vi "Start_Serving.vi"() -> ()   [LabVIEW 2022 SP3]
doc: "This is a simple example of a server which exports VIs to be called from another machine. You may run both the client.llb and server.llb on the same machine without modifying the access list. If you wish to run the client on another machine that is not in your domain you will have to list the name of the client in the Machine Access List. \n\nThe VIs listed in the Exported VI list are exported by the server.\n\nTo run this example start this VI First, then start the client.llb on all machines you want to try as clients. If you change either of the above lists, you must restart this VI for the changes to take effect.\n\nClick the \"Stop\" button to quit. This will turn off the server, terminating all client connections, and restore the previous access lists to their original values."
uses:
  Anemometry/Anemometry Sub Vis/Globals/Preference_global.vi
panel:
  out "logPath":path
  in  "Srvr.LogEnabled":bool
  out "Exported VI list":string[](array[string])
  # "These are the names of the VIs which will be allowed\nto be accessed from another machine."
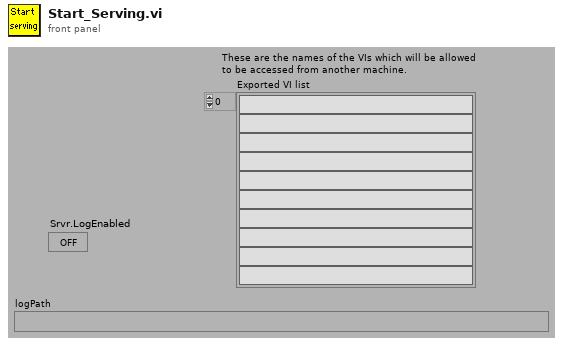
[diagram p1: front panel]
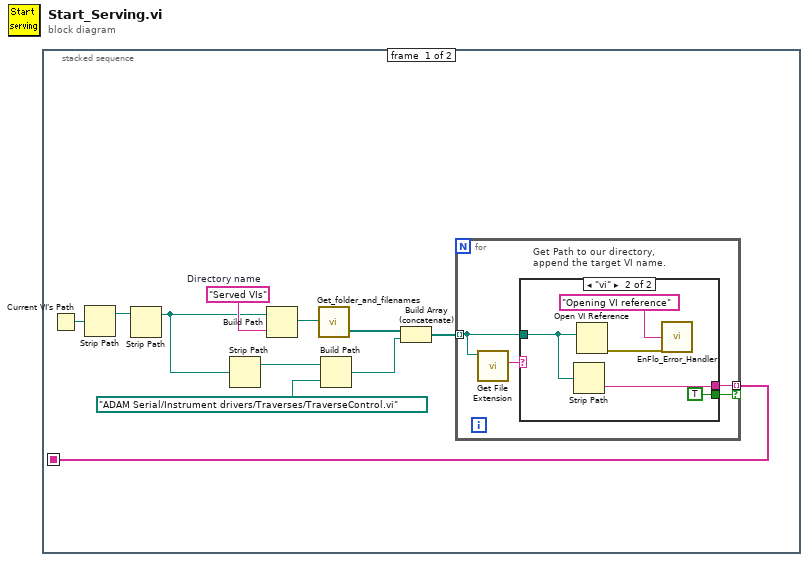
[diagram p0: block diagram]
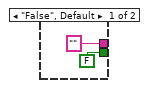
[diagram p2: hidden frame]
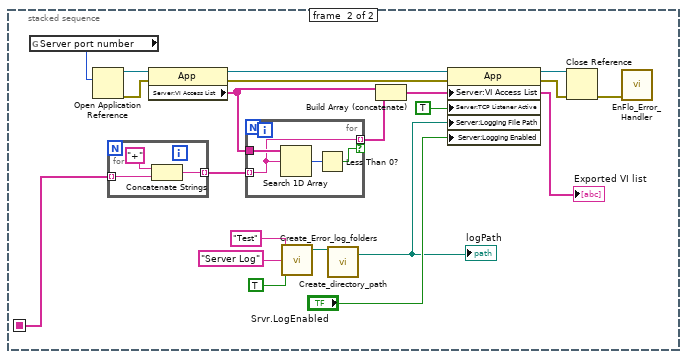
[diagram p3: hidden frame]
diagram:
  n1 = stacked-sequence {
    seq-local: [w1 _] -> [_ w26]
    frame #0 {
      w11 = "Served VIs"  # Directory name
      n2 = Current VI's Path() -> (path=w10:path)
      n3 = Strip Path(path=w10) -> (stripped path=w9:path)  [unwired: 1 out]
      n4 = Strip Path(path=w9) -> (stripped path=w7:path)  [unwired: 1 out]
      n5 = Strip Path(path=w7) -> (stripped path=w6:path)  [unwired: 1 out]
      n6 = Build Path(base path=w7, name or relative path=w11) -> (appended path=w8:path)
      n7 = call "Get_folder_and_filenames.vi"("file path (dialog if empty)"=w8) -> ("Files"=w4:path[])  [unwired: 1 out]
      n8 = Build Path(base path=w6, name or relative path=path "ADAM Serial/Instrument drivers/Traverses/TraverseControl.vi") -> (appended path=w3:path)
      n9 = Build Array (concatenate)(w4, w3) -> (w2:path[])
      n10 = for {
        tunnel: w2 -> [w14] mode=indexing
        tunnel: [w15] -> w1 mode=indexing if=w12
        # "Get Path to our directory,\nappend the target VI name."
        n11 = call <vilib>:"Get File Extension.vi"("file"=w14) -> ("lowercase file extension"=w13:string)  [unwired: 6 in, 4 out]
        n12 = case shown="\"vi\"" w13 {
          tunnel: ["" ("name") w22] -> w15
          tunnel: w14 -> [_ w19]
          tunnel: [FALSE TRUE] -> w12
          frame "False", Default {
          }
          frame "vi" {
            n13 = Strip Path(path=w19) -> (name=w22:string)  [unwired: 1 out]
            n14 = Open VI Reference(vi path=w19) -> (error out=w21:errorcluster)  [unwired: 2 in, 4 out]
            n15 = call "EnFlo_Error_Handler.vi"("error in (no error)"=w21, "Error Type"="Opening VI reference") -> ()  [unwired: 1 in, 3 out]
          }
        }
      }
    }
    frame #1 {
      n16 = global read "Preference_global.vi" "Server port number"() -> (w38:u32)
      n17 = Open Application Reference(10:w38) -> (0:w31:errorcluster, 3:w32:refnum<vi>)  [unwired: 1 in, 2 out]
      n18 = for {
        tunnel: [w44] -> w25 mode=indexing
        tunnel: w26 -> [w43] mode=indexing
        n19 = Concatenate Strings("+", w43) -> (w44:string)
      }
      n20 = property class="App"(reference=w32, error in=w31) -> (reference out=w30:refnum<vi>, error out=w29:errorcluster, "Server:VI Access List"=w28:string[])
      n21 = for {
        tunnel: w28 -> [w49]
        tunnel: w25 -> [w48] mode=indexing
        tunnel: [w48] -> w27 mode=indexing if=w46
        n22 = Search 1D Array(1D array=w49, element=w48) -> (index of element=w47:i32)  [unwired: 1 in]
        n23 = Less Than 0?(x=w47) -> (x < 0?=w46:bool)
      }
      n24 = call "Create_Error_log_folders.vi"("Log Filename"="Test", "Log Folder"="Server Log", "Per Day Log File?"=TRUE) -> ("Local Log File"=w33:path)  [unwired: 3 in, 1 out]
      n25 = call "Create_directory_path.vi"("Path name"=w33) -> ("Path name Out"=w24:path)  [unwired: 2 in, 1 out]
      "logPath" <- w24
      n26 = Build Array (concatenate)(w28, w27) -> (w23:string[])
      "Exported VI list" <- w23
      n27 = property class="App"(reference=w30, error in=w29, "Server:VI Access List"=w23, "Server:TCP Listener Active"=TRUE ("Srvr.TCPActive"), "Server:Logging File Path"=w24, "Server:Logging Enabled"="Srvr.LogEnabled") -> (reference out=w40:refnum<vi>, error out=w41:errorcluster)
      n28 = Close Reference(reference=w40, error in (no error)=w41) -> (error out=w42:errorcluster)
      n29 = call "EnFlo_Error_Handler.vi"("error in (no error)"=w42) -> ()  [unwired: 2 in, 3 out]
    }
  }
